vi "setPWM.vi"(8 "error in (no error)":errorcluster, 10 "PWM":u16, 11 "ISA010 in":refnum<class "ISA010.lvclass">) -> (0 "error out":errorcluster, 2 "Frame":string, 3 "ISA010 out":refnum<class "ISA010.lvclass">)   [LabVIEW 2017, in "ISA010.lvlib" / "ISA010.lvclass"]
uses:
  ISA010.lvclass
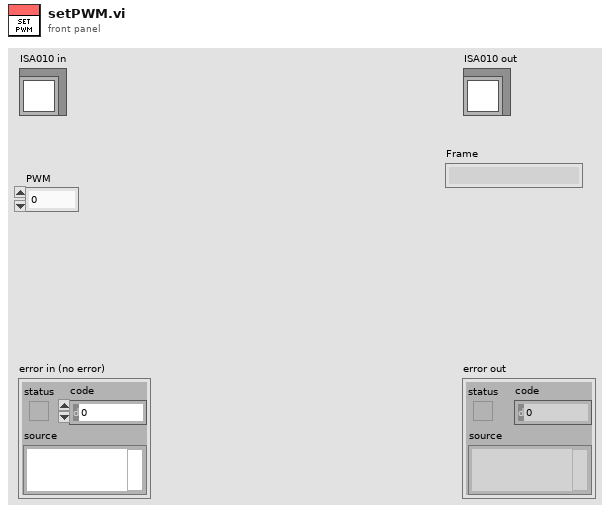
[diagram p1: front panel]
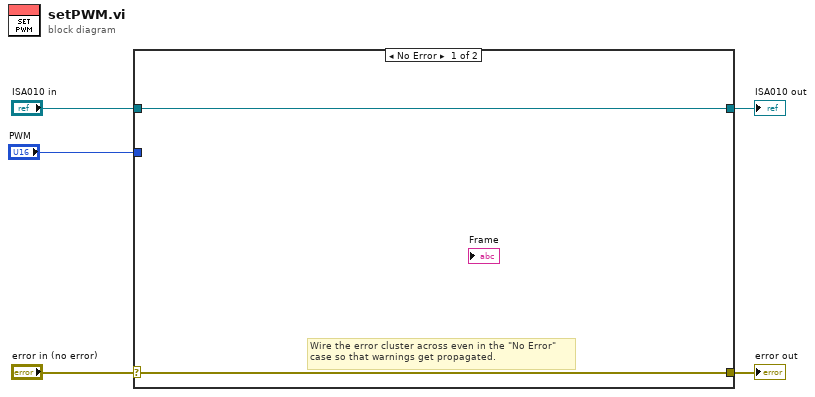
[diagram p0: block diagram]
diagram:
  n1 = case shown="No Error" "error in (no error)" {
    selector: "error in (no error)" -> [w6 w9]
    tunnel: [w6 w9] -> w4
    tunnel: [w7 w8] -> w2
    tunnel: "ISA010 in" -> [w7 w8]
    tunnel: "PWM" -> [_ _]
    frame No Error {
      # "Wire the error cluster across even in the \"No Error\"\ncase so that warnings get propagated."
    }
    frame Error {
    }
  }
  "error out" <- w4
  "ISA010 out" <- w2
